vi "get Property List.vi"(8 "error in":errorcluster, 9 "categoryName":string, 10 "resourceOrImageId":u32, 11 "cycloneHandle":u32) -> (0 "error out":errorcluster, 1 "categoryName out":string, 3 "function return":string)   [LabVIEW 2021, in "CycloneControlSDK.lvlib"]
doc: "extern \"C\" char * _cdecl getPropertyList(uint32_t cycloneHandle, uint32_t resourceOrImageId, char *categoryName);"
uses:
  CycloneControlSDK.lvlib
  CycloneControlSDK_64.dll
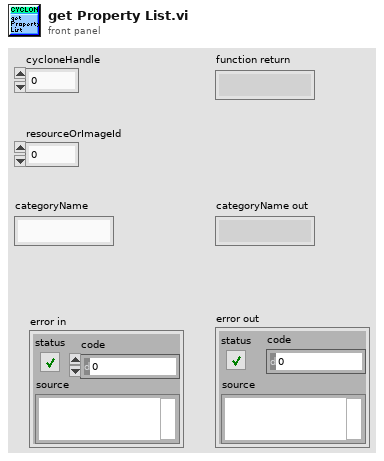
[diagram p1: front panel]
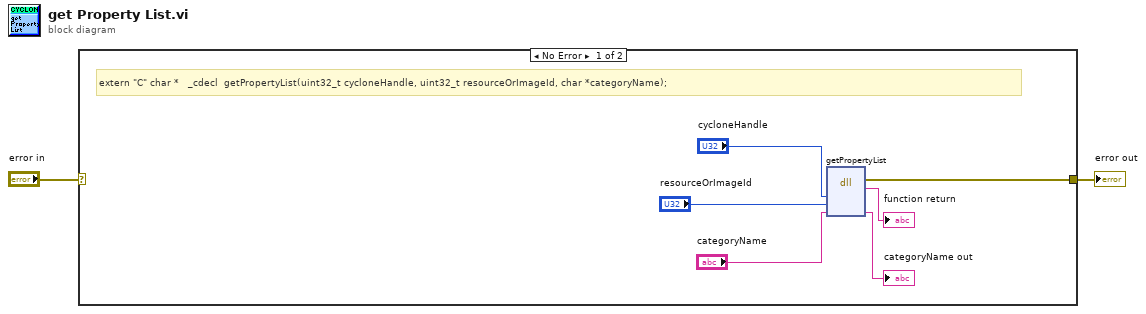
[diagram p0: block diagram]
diagram:
  n1 = case shown="No Error" "error in" {
    selector: "error in" -> [_ w9]
    tunnel: [w3 w9] -> w1
    frame No Error {
      # "extern \"C\" char *   _cdecl  getPropertyList(uint32_t cycloneHandle, uint32_t resourceOrImageId, char *categoryName);"
      n2 = dll-call lib="C:/PEMicro/cyclone/cycloneControl/controlsdk/examples/labview2018/user.lib/CycloneControlSDK/CycloneControlSDK_64.dll" fn="getPropertyList"("cycloneHandle"="cycloneHandle", "resourceOrImageId"="resourceOrImageId", "categoryName"="categoryName") -> (error out=w3:errorcluster, "return type"=→"function return":string, "categoryName"=→"categoryName out":string)  [unwired: 5 in, 1 out]
    }
    frame Error {
    }
  }
  "error out" <- w1
